vi "HandleJsonRpcRequest.vi"(8 "error in (no error)":errorcluster, 10 "Request":refnum<class "Request.lvclass">, 11 "SMO.jsonRPC":refnum<class "SMO.jsonRPC.lvclass">) -> (0 "error out":errorcluster, 2 "Response":refnum<class "Response.lvclass">, 3 "SMO.jsonRPC out":refnum<class "SMO.jsonRPC.lvclass">)   [LabVIEW 2013, in "SMO.jsonRPC.lvclass"]
doc: "---------------------------------------------------------------\nJKI State Machine Objects™\nhttp://jki.net/state-machine-objects/\nCopyright (C) 2005-2015, JKI <info@jki.net>\nALL RIGHTS RESERVEDJKI State Machine Objects (SMO) 1.0.0.5\nJKI - JKI\nCopyright (c) 2016, JKI"
uses:
  SMO.jsonRPC.lvclass
  <vilib>/JKI/JKI JSON RPC Specification/Request/Request.lvclass
  <vilib>/JKI/JKI JSON RPC Specification/Response/Response.lvclass
  <vilib>/JKI/JKI JSON RPC Specification/Request/Request.lvclass/Request.ctl
  <vilib>/JKI/JKI JSON RPC Specification/Error/JSON-RPC Error Codes.ctl
  <vilib>/Utility/VariantDataType/GetTypeInfo.vi
  <vilib>/JKI/JKI JSON RPC Specification/Error/Error.lvclass
  <vilib>/addons/_JKI.lib/Serialization/JSON/JKI JSON Serialization.lvlib
panel:
  # "For instructions on how to use the JKI State Machine Objects, examples and video tutorials, visit:\nhttp://jki.net/state-machine-objects/\n\nJKI State Machine Objects™\nhttp://jki.net/state-machine-objects/\nCopyright (C) 2005-2015, JKI <info@jki.net>\nALL RIGHTS RESERVED"
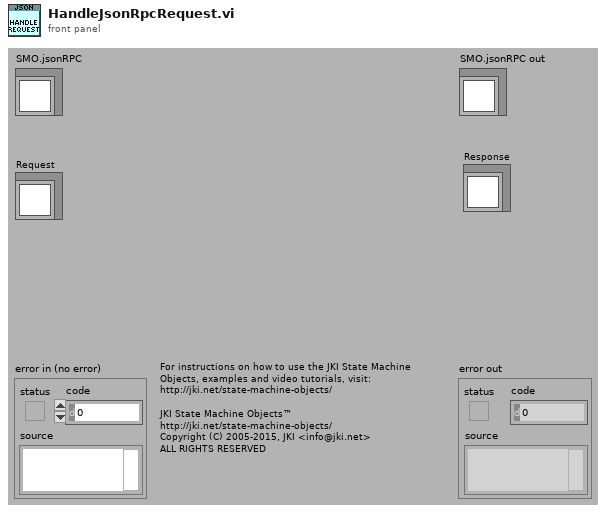
[diagram p1: front panel]
types:
  T1 = typedef "JSON RPC 2.0.lvlib/Error.lvclass/JSON-RPC Error Codes.ctl" = i16
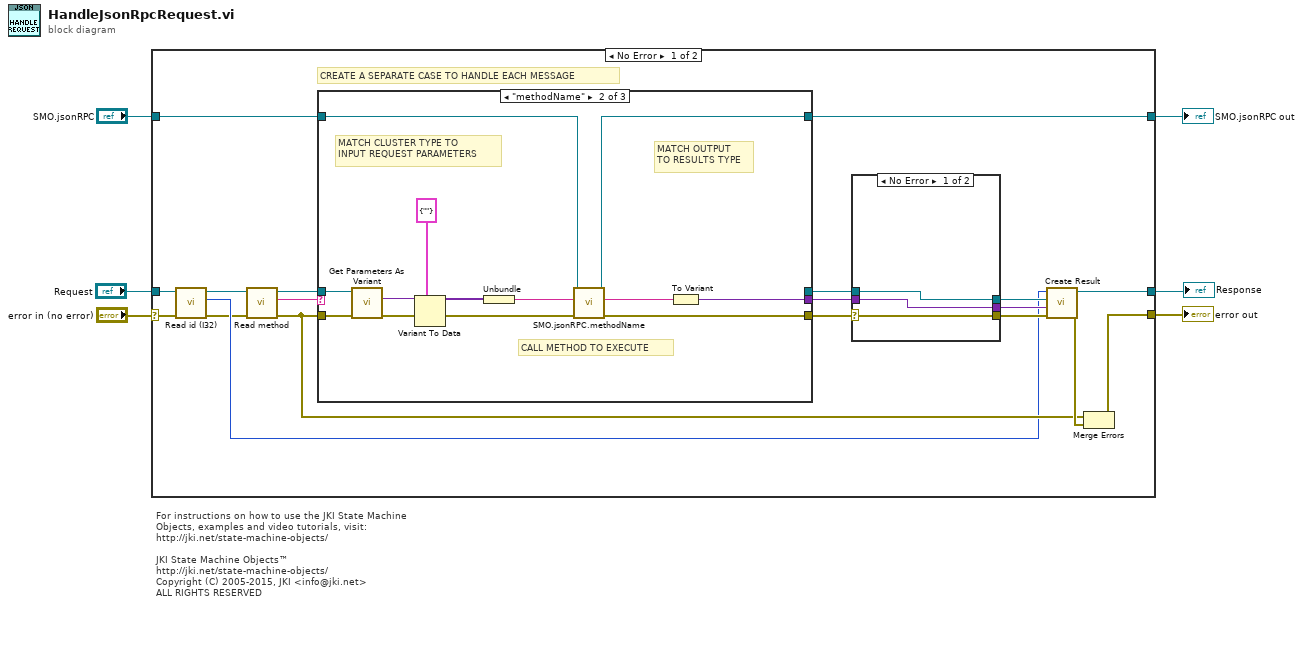
[diagram p0: block diagram]
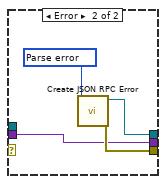
[diagram p2: hidden frame]
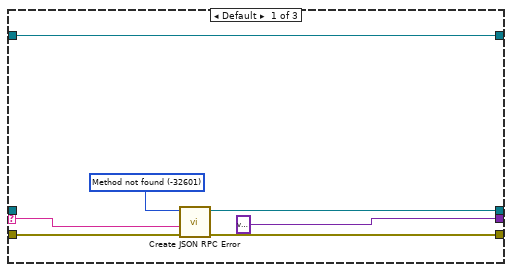
[diagram p3: hidden frame]
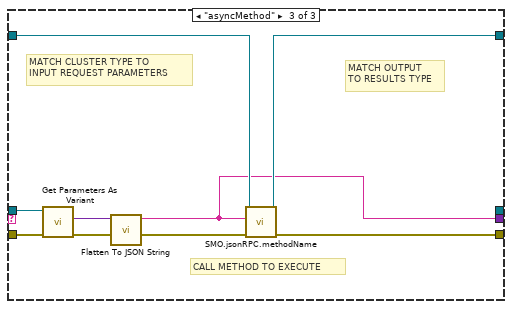
[diagram p4: hidden frame]
diagram:
  # "For instructions on how to use the JKI State Machine Objects, examples and video tutorials, visit:\nhttp://jki.net/state-machine-objects/\n\nJKI State Machine Objects™\nhttp://jki.net/state-machine-objects/\nCopyright (C) 2005-2015, JKI <info@jki.net>\nALL RIGHTS RESERVED"
  n1 = case shown="No Error" "error in (no error)" {
    selector: "error in (no error)" -> [w9 w62]
    tunnel: "SMO.jsonRPC" -> [w25 w63]
    tunnel: [w16 w62] -> w5
    tunnel: [w24 w63] -> w4
    tunnel: "Request" -> [w11 _]
    tunnel: [w17 _] -> w1
    frame No Error {
      # "CREATE A SEPARATE CASE TO HANDLE EACH MESSAGE"
      n2 = call <vilib>:"Read id (I32).vi"("error in (no error)"=w9, "Request in"=w11) -> ("error out"=w8:errorcluster, "id"=w10:i32, "Request out"=w7:refnum<class "Request.lvclass">)  [unwired: 7 in]
      n3 = call <vilib>:"Read method.vi"("error in (no error)"=w8, "Request in"=w7) -> ("error out"=w15:errorcluster, "method"=w22:string, "Request out"=w23:refnum<class "Request.lvclass">)  [unwired: 7 in]
      n4 = case shown="\"methodName\"" w22 {
        selector: w22 -> [w33 _ _]
        tunnel: w25 -> [w39 w45 w59]
        tunnel: [w36 w40 w54] -> w20
        tunnel: [w39 w44 w58] -> w24
        tunnel: w23 -> [_ w52 w61]
        tunnel: w15 -> [w37 w50 w60]
        tunnel: [variant ("Variant") w41 w53] -> w19
        tunnel: [w35 _ _] -> w18
        frame Default {
          w38 = T1 -32601 items=["Parse error"=-32700, "Internal error"=-32603, "Invalid params"=-32602, "Method not found"=-32601, "Invalid Request"=-32600] ("JSON RPC Error")
          n5 = call <vilib>:"Create JSON RPC Error.vi"("error in (no error)"=w37, "data"=w33, "JSON RPC Error"=w38) -> ("error out"=w36:errorcluster, "Error out"=w35:refnum<class "Error.lvclass">)  [unwired: 6 in, 1 out]
        }
        frame "methodName" {
          # "CALL METHOD TO EXECUTE"
          # "MATCH OUTPUT\nTO RESULTS TYPE"
          # "MATCH CLUSTER TYPE TO\nINPUT REQUEST PARAMETERS"
          n6 = call <vilib>:"Get Parameters As Variant.vi"("error in (no error)"=w50, "Request in"=w52) -> ("error out"=w43:errorcluster, "params"=w51:variant)  [unwired: 7 in, 1 out]
          n7 = Variant To Data(error in=w43, type=cluster{string} {""}, Variant=w51) -> (data=w49:cluster{string}, error out=w42:errorcluster)
          n8 = Unbundle(w49) -> (w47:string)
          n9 = call "SMO.jsonRPC.methodName.vi"("error in (no error)"=w42, "myData"=w47, "SMO.ByRefWithEvents"=w45) -> ("error out"=w40:errorcluster, "Data Out"=w46:string, "SMO.ByRefWithEvents out"=w44:refnum<class "SMO.jsonRPC.lvclass">)  [unwired: 6 in]
          n10 = To Variant(anything=w46) -> (Variant=w41:variant)
        }
        frame "asyncMethod" {
          # "CALL METHOD TO EXECUTE"
          # "MATCH OUTPUT\nTO RESULTS TYPE"
          # "MATCH CLUSTER TYPE TO\nINPUT REQUEST PARAMETERS"
          n11 = call <vilib>:"Get Parameters As Variant.vi"("error in (no error)"=w60, "Request in"=w61) -> ("error out"=w56:errorcluster, "params"=w57:variant)  [unwired: 7 in, 1 out]
          n12 = call <vilib>:"Flatten To JSON String.vi"("error in (no error)"=w56, "Variant"=w57) -> ("error out"=w55:errorcluster, "JSON String"=w53:string)  [unwired: 8 in]
          n13 = call "SMO.jsonRPC.methodName.vi"("error in (no error)"=w55, "myData"=w53, "SMO.ByRefWithEvents"=w59) -> ("error out"=w54:errorcluster, "SMO.ByRefWithEvents out"=w58:refnum<class "SMO.jsonRPC.lvclass">)  [unwired: 6 in, 1 out]
        }
      }
      n14 = case shown="No Error" w20 {
        selector: w20 -> [w27 _]
        tunnel: w19 -> [w26 w29]
        tunnel: w18 -> [w28 _]
        tunnel: [w28 w31] -> w14
        tunnel: [w27 w30] -> w13
        tunnel: [w26 w29] -> w12
        frame No Error {
        }
        frame Error {
          w32 = T1 -32700 items=["Parse error"=-32700, "Internal error"=-32603, "Invalid params"=-32602, "Method not found"=-32601, "Invalid Request"=-32600] ("JSON RPC Error")
          n15 = call <vilib>:"Create JSON RPC Error.vi"("JSON RPC Error"=w32) -> ("error out"=w30:errorcluster, "Error out"=w31:refnum<class "Error.lvclass">)  [unwired: 8 in, 1 out]
        }
      }
      n16 = call <vilib>:"Create Result.vi"("error in (no error)"=w13, "result"=w12, "Error"=w14, "id (-1: notification)"=w10) -> ("error out"=w21:errorcluster, "Response"=w17:refnum<class "Response.lvclass">)  [unwired: 5 in, 1 out]
      n17 = Merge Errors(w15, w21) -> (w16:errorcluster)
    }
    frame Error {
    }
  }
  "error out" <- w5
  "SMO.jsonRPC out" <- w4
  "Response" <- w1
